vi "S2C_InstrOpen.vi"(8 "Error In":errorcluster) -> (0 "Error Out":errorcluster)   [LabVIEW 2015]
doc: "Opens a connection to all instruments and launches the Fornax process."
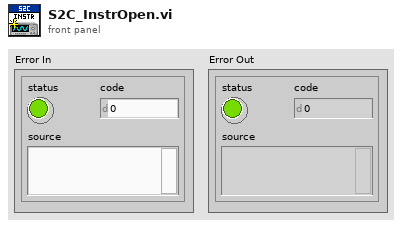
[diagram p1: front panel]
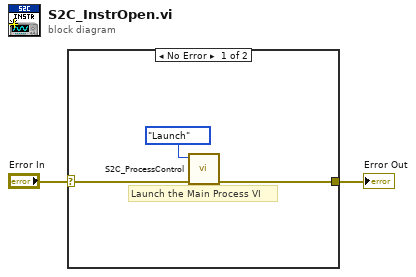
[diagram p0: block diagram]
diagram:
  n1 = case shown="No Error" "Error In" {
    selector: "Error In" -> [w3 w6]
    tunnel: [w4 w6] -> w2
    frame No Error {
      # "Launch the Main Process VI"
      n2 = call "S2C_ProcessControl.vi"("Error In"=w3, "Action"=enum16{"Launch", "Exit"}."Launch") -> ("Error Out"=w4:errorcluster)  [unwired: 9 in]
    }
    frame Error {
    }
  }
  "Error Out" <- w2
